vi "Destroy Class.vi"(8 "error in (no error)":errorcluster, 11 "Process State":refnum<data-value>) -> (0 "error out":errorcluster)   [LabVIEW 2022 SP3, in "Process State Data.lvclass"]
uses:
  Process State Data.lvclass
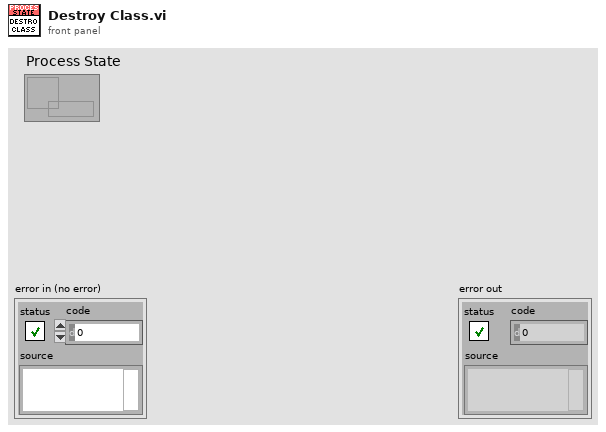
[diagram p1: front panel]
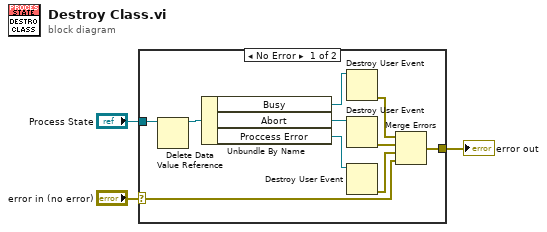
[diagram p0: block diagram]
diagram:
  n1 = case shown="No Error" "error in (no error)" {
    selector: "error in (no error)" -> [w13 w14]
    tunnel: [w7 w14] -> w2
    tunnel: "Process State" -> [w12 _]
    frame No Error {
      n2 = Delete Data Value Reference(data value reference=w12) -> (data value=w11:refnum<class "Process State Data.lvclass">)  [unwired: 1 in, 1 out]
      n3 = Unbundle By Name(w11) -> ("Busy"=w10:refnum<user-event>, "Abort"=w9:refnum<user-event>, "Proccess Error"=w8:refnum<user-event>)
      n4 = Destroy User Event(user event=w10) -> (error out=w6:errorcluster)  [unwired: 1 in]
      n5 = Destroy User Event(user event=w9) -> (error out=w5:errorcluster)  [unwired: 1 in]
      n6 = Destroy User Event(user event=w8) -> (error out=w4:errorcluster)  [unwired: 1 in]
      n7 = Merge Errors(w6, w5, w4, w13) -> (w7:errorcluster)
    }
    frame Error {
    }
  }
  "error out" <- w2
